vi "Wait for Running.vi"(7 "Timeout (10s)":dbl=10.0, 8 "error in (no error)":errorcluster, 10 "Running":bool, 11 "Panel in":refnum<class "Panel.lvclass">) -> (0 "error out":errorcluster, 3 "Panel out":refnum<class "Panel.lvclass">)   [LabVIEW 2020, in "OOPanel.lvlib" / "Panel.lvclass"]
uses:
  Panel.lvclass
  Panel.lvclass/Panel.ctl
  <vilib>/Utility/error.llb/Error Cluster From Error Code.vi
  <vilib>/ErrorRing/Error Ring.xnode
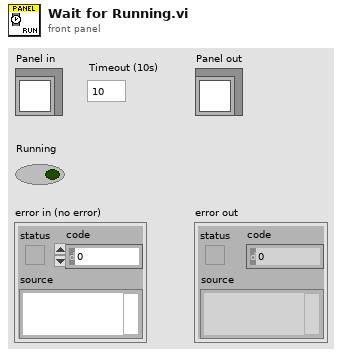
[diagram p1: front panel]
types:
  T1 = typedef "OOPanel.lvlib/Panel.lvclass/Ref Data.ctl" = cluster{"Panel Events":T2, "Panel Ref":refnum<vi>, "SubPanel":refnum<vi>, "Close":bool, "Running":bool, "State":T3}
  T2 = typedef "OOPanel.lvlib/Panel.lvclass/Panel Events.ctl" = cluster{"Visbility":refnum<user-event>, "Close":refnum<user-event>}
  T3 = typedef "OOPanel.lvlib/Panel.lvclass/Visibility State.ctl" = enum16{"Idle", "Closed", "Hidden", "Visible", "Subpanel"}
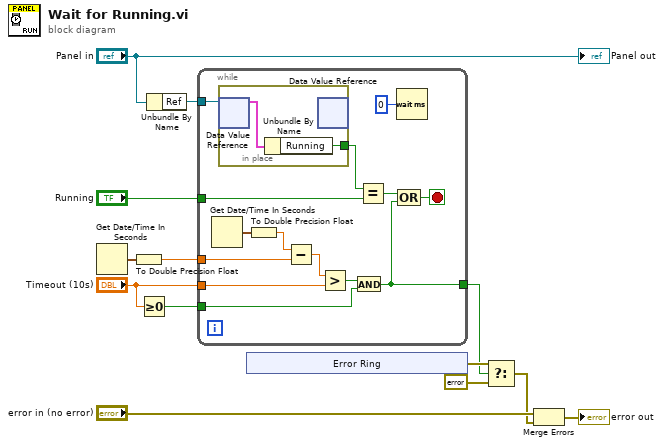
[diagram p0: block diagram]
diagram:
  n1 = Get Date/Time In Seconds() -> (seconds since 1Jan1904=w12:timestamp)
  n2 = To Double Precision Float(number=w12) -> (double precision float=w9:dbl)
  n3 = Greater Or Equal To 0?(x="Timeout (10s)") -> (x >= 0?=w6:bool)
  n4 = Unbundle By Name("Panel in") -> ("Ref"=w11:refnum<data-value>)
  n5 = while {
    tunnel: w11 -> [w27]
    tunnel: w9 -> [w25]
    tunnel: "Running" -> [w21]
    tunnel: "Timeout (10s)" -> [w23]
    tunnel: w6 -> [w16]
    tunnel: [w14] -> w4
    stop <- w18 stop-if-true
    n6 = Get Date/Time In Seconds() -> (seconds since 1Jan1904=w26:timestamp)
    n7 = in-place {
      in-place-border: [w28] -> w20
      n8 = in-place-dvr #1(w27) -> (w29:T1)  [unwired: 1 out]
      n9 = Unbundle By Name(w29) -> ("Running"=w28:bool)
      n10 = in-place-dvr #1() -> ()  [unwired: 1 in, 2 out]
    }
    n11 = To Double Precision Float(number=w26) -> (double precision float=w24:dbl)
    n12 = Subtract(x=w24, y=w25) -> (x-y=w22:dbl)
    n13 = Greater?(x=w22, y=w23) -> (0:w17:bool)
    n14 = And(x=w17, y=w16) -> (x .and. y?=w14:bool)
    n15 = Equal?(x=w20, y=w21) -> (x = y?=w19:bool)
    n16 = Wait (ms)(milliseconds to wait=u32 0) -> ()  [unwired: 1 out]
    n17 = Compound Arithmetic op=OR(w19, w14) -> (w18:bool)
  }
  n18 = xnode "Error Ring"() -> ("error out"=w5:errorcluster)
  n19 = Select(t=w5, s=w4, f=errorcluster {"status"=FALSE, "code"=0, "source"=""}) -> (s? t:f=w1:errorcluster)
  n20 = Merge Errors("error in (no error)", w1) -> (→"error out":errorcluster)
  "Panel out" <- "Panel in"
